vi "Expand Channel Names.vi"(10 "Group Names":string[](array[string]), 11 "Channels":string[](array[string])) -> (3 "Channel Names":string[](array[string]))   [LabVIEW 2013]
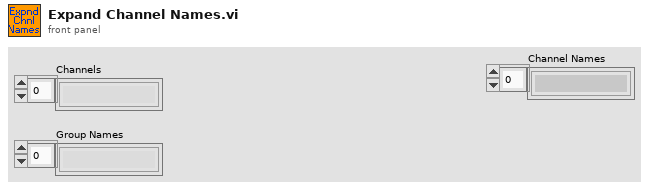
[diagram p1: front panel]
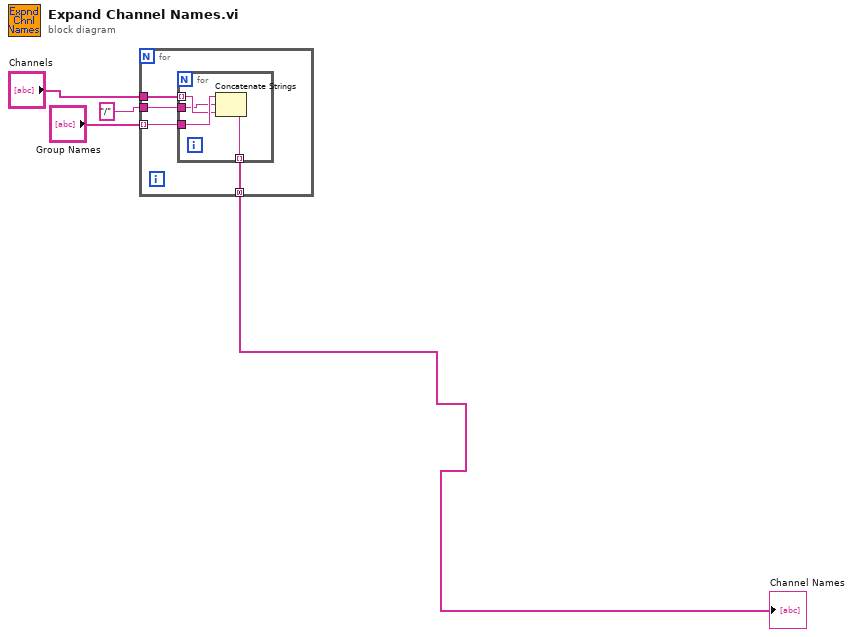
[diagram p0: block diagram]
diagram:
  n1 = for {
    tunnel: "Channels" -> [w8]
    tunnel: "Group Names" -> [w7] mode=indexing
    tunnel: "/" ("string") -> [w6]
    tunnel: [w5] -> w4 mode=concatenating
    n2 = for {
      tunnel: w8 -> [w11] mode=indexing
      tunnel: w7 -> [w12]
      tunnel: w6 -> [w10]
      tunnel: [w9] -> w5 mode=indexing
      n3 = Concatenate Strings(w12, w10, w11) -> (w9:string)
    }
  }
  "Channel Names" <- w4
